vi "Scint2HitchartClustIndex.vi"(11 "Channel":i8) -> (3 "Numeric":i8)   [LabVIEW 2016]
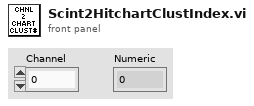
[diagram p1: front panel]
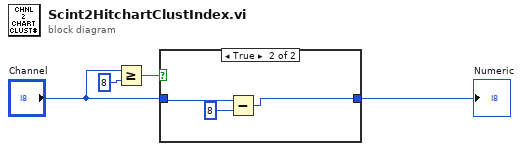
[diagram p0: block diagram]
diagram:
  n1 = Greater Or Equal?(x="Channel", y=i8 8) -> (x >= y?=w2:bool)
  n2 = case shown="True" w2 {
    tunnel: "Channel" -> [w5 w8]
    tunnel: [w5 w6] -> w1
    frame False {
    }
    frame True {
      n3 = Subtract(x=w8, y=i8 8) -> (x-y=w6:i8)
    }
  }
  "Numeric" <- w1
